vi "Get Temperature.vi"   [LabVIEW 2013, in "LVH-Nest.lvlib"]
doc: "Read the current temperature from specified Nest device."
uses:
  LVH-Nest.lvlib
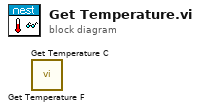
[diagram p0: block diagram]
diagram:
  n1 = call "Get Temperature F.vi"() -> ()  [unwired: 9 in, 3 out]
  n2 = call "Get Temperature C.vi"() -> ()  [unwired: 9 in, 3 out]
